vi "Init Game.vi"(8 "error in":errorcluster, 11 "Game in":refnum<class "Game.lvclass">) -> (0 "error out":errorcluster, 3 "Game out":refnum<class "Game.lvclass">)   [LabVIEW 2021, in "Game.lvclass"]
uses:
  Game.lvclass
  Game.lvclass/Game.ctl
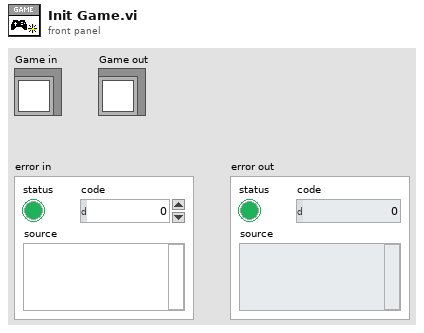
[diagram p1: front panel]
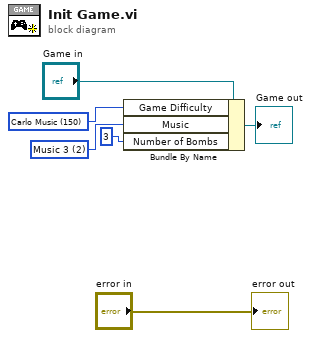
[diagram p0: block diagram]
diagram:
  w4 = u32 2 items=["Music 1", "Music 2", "Music 3", "Music 4"] ("Music:")
  w3 = u32 150 items=["Easy"=750, "Hard"=500, "Extreme"=300, "Carlo Music"=150] ("Game Difficulty:")
  n1 = Bundle By Name(cluster="Game in", "Game Difficulty"=w3, "Music"=w4, "Number of Bombs"=3) -> (→"Game out":refnum<class "Game.lvclass">)
  "error out" <- "error in"
